vi "Do.vi"(8 "error in (no error)":errorcluster, 10 "\"this\" object in":variant, 11 "AppLogger.Message.Log in":refnum<class "AppLogger.Message.Log.lvclass">) -> (0 "error out":errorcluster, 3 "AppLogger.Message.Log out":refnum<class "AppLogger.Message.Log.lvclass">)   [LabVIEW 2014, in "AppLogger.Message.Log.lvclass"]
uses:
  AppLogger.Message.Log.lvclass
  AppLogger.lvclass
  AppLogger.Message.Log.lvclass/AppLogger.Message.Log.ctl
panel:
  in  "AppLogger.lvclass":refnum<class "AppLogger.lvclass">
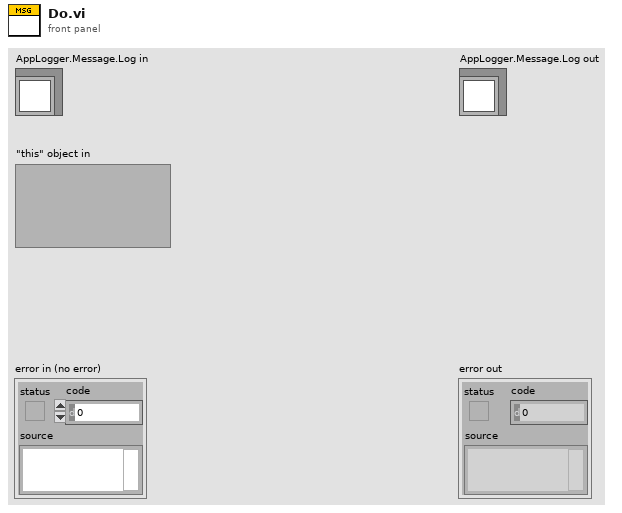
[diagram p1: front panel]
types:
  T1 = typedef "AppLogger.Message.Log.lvclass/Enum.LogLevel.ctl" = enum16{"Info", "Warning", "Small Error", "Fatal Error"}
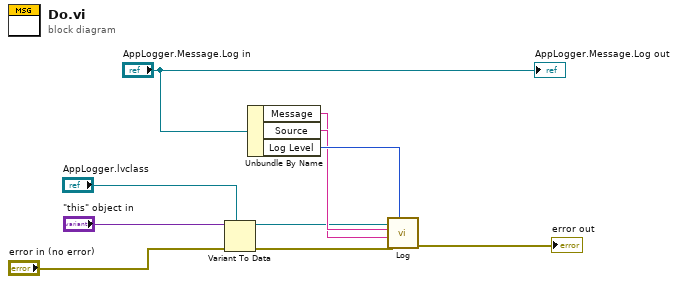
[diagram p0: block diagram]
diagram:
  n1 = Variant To Data(error in="error in (no error)", type="AppLogger.lvclass", Variant="\"this\" object in") -> (data=w1:refnum<class "AppLogger.lvclass">, error out=w2:errorcluster)
  n2 = Unbundle By Name("AppLogger.Message.Log in") -> ("Message"=w7:string, "Source"=w8:string, "Log Level"=w9:T1)
  n3 = call "Log.vi"("Log Level"=w9, "error in (no error)"=w2, "Message"=w7, "Source"=w8, "AppLogger in"=w1) -> ("error out"=→"error out":errorcluster)  [unwired: 5 in, 1 out]
  "AppLogger.Message.Log out" <- "AppLogger.Message.Log in"
